vi "Teleop - Toggle (SubVI).vi"(11 "Value In":bool) -> (3 "Toggle out":bool)   [LabVIEW 2019]
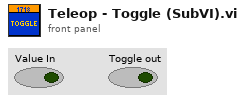
[diagram p1: front panel]
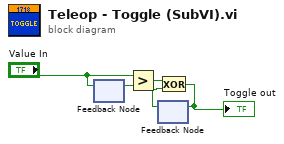
[diagram p0: block diagram]
diagram:
  n1 = feedback #1() -> (w4:bool)  [unwired: 1 in]
  n2 = feedback-in #1("Value In") -> ()
  n3 = Greater?(x="Value In", y=w4) -> (0:w3:bool)
  n4 = feedback #2() -> (w2:bool)  [unwired: 1 in]
  n5 = Exclusive Or(1:w2, 2:w3) -> (0:w1:bool)
  "Toggle out" <- w1
  n6 = feedback-in #2(w1) -> ()
